vi "Fix Resource Size Bytes.vi"(1 "Data In":string) -> (0 "Data Out":string)   [LabVIEW 2017]
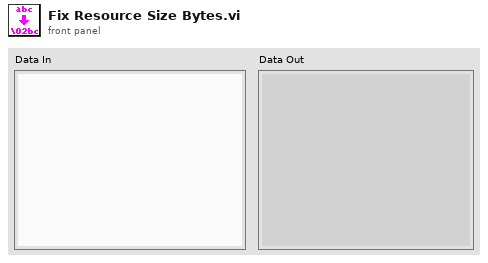
[diagram p1: front panel]
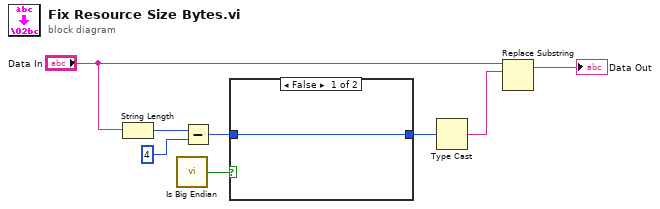
[diagram p0: block diagram]
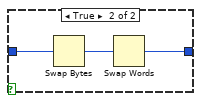
[diagram p2: hidden frame]
diagram:
  n1 = String Length(string="Data In") -> (length=w2:i32)
  n2 = call "Is Big Endian.vi"() -> ("big endian"=w7:bool)
  n3 = Subtract(x=w2, y=4) -> (x-y=w3:i32)
  n4 = case shown="False" w7 {
    tunnel: [w9 w11] -> w6
    tunnel: w3 -> [w9 w10]
    frame False {
    }
    frame True {
      n5 = Swap Bytes(anything=w10) -> (byte swapped=w12:i32)
      n6 = Swap Words(1:w12) -> (0:w11:i32)
    }
  }
  n7 = Type Cast(x=w6) -> (*(type *) &x=w5:string)  [unwired: 1 in]
  n8 = Replace Substring(4:w5, 5:"Data In") -> (1:→"Data Out":string)  [unwired: 2 in, 1 out]
